vi "BLM_stepper motor V2.vi"() -> ()   [LabVIEW 2018]
doc: "To start rotations:\n\nSelect The Motor (BLM) address\nRun this VI\nClick Test connection button\nClick INITIALIZE button \n (It is assumed that a BLM controller should be initialized only once: immediately after it is turned on. \n E.g., usually there is no need to initialize if you rebooted computer, but kept the motor controller on,\n the motor was connected to the controller and you wish to continue using current position counting. \n Initialization occurs only if the current motor position is equal to zero.) \nClick READ BLM position button\nSelect desired MODE, SPEED, and Distance (or Final Position, depends on the MODE) value\nClick RUN BLM button\n\nSET POSITION button does not affect actual sample/motor position, but changes the position value\nin the controller memory. Thus, it allows to assign any value to the current motor position.\n\nSee also:\nhttps://opswiki.magnet.fsu.edu/wiki/pages/K7Q8u4C4s9/Rotating_probes_equipped_with_Brushless_Motors_BLMs.html\n\nNHMFL; A.Suslov; Feb 2012; updated Aug 2016"
uses:
  stepper motor action.ctl
  slider setter action.ctl
  stepper motor state.ctl
panel:
  in  "Tab Control":enum32{"main", "init&stuff", "ignore"}(tab)
  in  "stepper state":T1=enum."stopped"
  in  "set angle":dbl(slide)=-18.244680851063833 scale=-95.0..95.0 scale format="%^#6_6g"
  in  "XY Graph":cluster{dbl[], dbl[]}[](graph)=[{[-0.2849184585575504, -0.22366098996767705, -0.16240352137780373, -0.10114605278793037, -0.03988858419805705, 0.02136888439181628, 0.08262635298168963, 0.14388382157156293, 0.20514129016143628, 0.2663987587513096, 0.32765622734118294, 0.3889136959310563, 0.45017116452092965, 0.511428633110803, 0.5726861017006762, 0.6339435702905496, 0.695201038880423, 0.7564585074702963, 0.8177159760601695, 0.878973444650043], [0.09392269147117449, 0.07372931280487197, 0.053535934138569455, 0.03334255547226694, 0.013149176805964419, -0.007044201860338106, -0.027237580526640617, -0.04743095919294313, -0.06762433785924565, -0.08781771652554818, -0.1080110951918507, -0.1282044738581532, -0.14839785252445573, -0.16859123119075825, -0.18878460985706075, -0.2089779885233633, -0.2291713671896658, -0.2493647458559683, -0.26955812452227085, -0.28975150318857334]}, {[0.02614672282429747, 0.020525177417073513, 0.014903632009849559, 0.0092820866026256, 0.003660541195401646, -0.0019610042118223085, -0.00758254961904627, -0.013204095026270225, -0.01882564043349418, -0.024447185840718134, -0.03006873124794209, -0.03569027665516605, -0.04131182206239001, -0.04693336746961396, -0.05255491287683792, -0.05817645828406187, -0.06379800369128583, -0.06941954909850978, -0.07504109450573374, -0.08066263991295769], [0.2988584094275236, 0.23460385140060602, 0.17034929337368845, 0.10609473534677089, 0.04184017731985329, -0.022414380707064308, -0.08666893873398185, -0.15092349676089944, -0.21517805478781704, -0.27943261281473464, -0.34368717084165223, -0.40794172886856983, -0.4721962868954873, -0.5364508449224049, -0.6007054029493225, -0.6649599609762401, -0.7292145190031577, -0.7934690770300753, -0.8577236350569929, -0.9219781930839105]}, {[1.0, 0.9980267284282716, 0.9921147013144779, 0.9822872507286887, 0.9685831611286311, 0.9510565162951535, 0.9297764858882513, 0.9048270524660195, 0.8763066800438636, 0.8443279255020151, 0.8090169943749475, 0.7705132427757891, 0.7289686274214116, 0.6845471059286886, 0.6374239897486896, 0.587785252292473, 0.5358267949789965, 0.48175367410171516, 0.42577929156507266, 0.36812455268467786, 0.30901699437494745, 0.24868988716485474, 0.18738131458572452, 0.12533323356430426, 0.0627905195293133, -1.6081428723391245e-16, -0.0627905195293134, -0.12533323356430437, -0.18738131458572482, -0.24868988716485485, -0.30901699437494756, -0.368124552684678, -0.4257792915650727, -0.48175367410171543, -0.5358267949789969, -0.587785252292473, -0.6374239897486897, -0.6845471059286887, -0.7289686274214117, -0.7705132427757894, -0.8090169943749473, -0.8443279255020151, -0.8763066800438636, -0.9048270524660196, -0.9297764858882515, -0.9510565162951536, -0.9685831611286311, -0.9822872507286887, -0.9921147013144779, -0.9980267284282716, -1.0, -0.9980267284282716, -0.9921147013144779, -0.9822872507286886, -0.9685831611286311, -0.9510565162951535, -0.9297764858882512, -0.9048270524660195, -0.8763066800438635, -0.844327925502015, -0.8090169943749472, -0.770513242775789, -0.7289686274214116, -0.6845471059286886, -0.6374239897486895, -0.5877852522924732, -0.5358267949789963, -0.48175367410171527, -0.42577929156507216, -0.3681245526846778, -0.30901699437494756, -0.24868988716485443, -0.18738131458572463, -0.12533323356430373, -0.06279051952931321, -1.836909530733566e-16, 0.06279051952931372, 0.12533323356430423, 0.18738131458572513, 0.24868988716485493, 0.30901699437494723, 0.36812455268467825, 0.4257792915650726, 0.4817536741017157, 0.5358267949789968, 0.5877852522924737, 0.63742398974869, 0.6845471059286886, 0.7289686274214119, 0.7705132427757894, 0.8090169943749478, 0.8443279255020153, 0.8763066800438636, 0.9048270524660197, 0.9297764858882515, 0.9510565162951538, 0.9685831611286312, 0.9822872507286887, 0.9921147013144779, 0.9980267284282716], [0.0, 0.06279051952931337, 0.12533323356430426, 0.18738131458572463, 0.2486898871648548, 0.3090169943749474, 0.368124552684678, 0.4257792915650727, 0.4817536741017153, 0.5358267949789967, 0.5877852522924731, 0.6374239897486897, 0.6845471059286887, 0.7289686274214116, 0.7705132427757893, 0.8090169943749475, 0.8443279255020151, 0.8763066800438637, 0.9048270524660196, 0.9297764858882515, 0.9510565162951535, 0.9685831611286311, 0.9822872507286887, 0.9921147013144779, 0.9980267284282716, 1.0, 0.9980267284282716, 0.9921147013144778, 0.9822872507286886, 0.9685831611286311, 0.9510565162951535, 0.9297764858882513, 0.9048270524660195, 0.8763066800438635, 0.844327925502015, 0.8090169943749475, 0.7705132427757893, 0.7289686274214114, 0.6845471059286885, 0.6374239897486895, 0.5877852522924732, 0.5358267949789967, 0.4817536741017152, 0.4257792915650725, 0.36812455268467775, 0.3090169943749471, 0.24868988716485482, 0.18738131458572457, 0.1253332335643041, 0.06279051952931314, -3.216285744678249e-16, -0.06279051952931335, -0.12533323356430429, -0.18738131458572477, -0.24868988716485502, -0.30901699437494773, -0.3681245526846783, -0.42577929156507266, -0.4817536741017154, -0.5358267949789968, -0.5877852522924734, -0.63742398974869, -0.6845471059286887, -0.7289686274214116, -0.7705132427757894, -0.8090169943749473, -0.8443279255020153, -0.8763066800438636, -0.9048270524660198, -0.9297764858882515, -0.9510565162951535, -0.9685831611286312, -0.9822872507286887, -0.9921147013144779, -0.9980267284282716, -1.0, -0.9980267284282716, -0.9921147013144779, -0.9822872507286886, -0.9685831611286311, -0.9510565162951536, -0.9297764858882512, -0.9048270524660196, -0.8763066800438634, -0.844327925502015, -0.809016994374947, -0.770513242775789, -0.7289686274214116, -0.6845471059286883, -0.6374239897486896, -0.5877852522924726, -0.5358267949789963, -0.4817536741017153, -0.4257792915650722, -0.36812455268467786, -0.3090169943749468, -0.2486898871648545, -0.18738131458572468, -0.1253332335643038, -0.06279051952931326]}, {[0.1, 0.09980267284282716, 0.0992114701314478, 0.09822872507286888, 0.09685831611286311, 0.09510565162951536, 0.09297764858882514, 0.09048270524660196, 0.08763066800438636, 0.08443279255020152, 0.08090169943749476, 0.07705132427757892, 0.07289686274214116, 0.06845471059286887, 0.06374239897486897, 0.05877852522924731, 0.05358267949789966, 0.04817536741017152, 0.042577929156507266, 0.03681245526846779, 0.030901699437494747, 0.024868988716485477, 0.018738131458572452, 0.012533323356430426, 0.006279051952931331, -1.6081428723391246e-17, -0.0062790519529313405, -0.012533323356430438, -0.018738131458572484, -0.024868988716485487, -0.030901699437494757, -0.0368124552684678, -0.04257792915650727, -0.048175367410171546, -0.05358267949789969, -0.05877852522924731, -0.06374239897486898, -0.06845471059286888, -0.07289686274214117, -0.07705132427757894, -0.08090169943749474, -0.08443279255020152, -0.08763066800438636, -0.09048270524660196, -0.09297764858882515, -0.09510565162951537, -0.09685831611286311, -0.09822872507286888, -0.0992114701314478, -0.09980267284282716, -0.1, -0.09980267284282716, -0.0992114701314478, -0.09822872507286887, -0.09685831611286311, -0.09510565162951536, -0.09297764858882512, -0.09048270524660196, -0.08763066800438635, -0.0844327925502015, -0.08090169943749473, -0.07705132427757891, -0.07289686274214116, -0.06845471059286887, -0.06374239897486896, -0.05877852522924733, -0.05358267949789963, -0.04817536741017153, -0.04257792915650722, -0.036812455268467784, -0.030901699437494757, -0.024868988716485445, -0.018738131458572463, -0.012533323356430374, -0.006279051952931321, -1.836909530733566e-17, 0.006279051952931373, 0.012533323356430424, 0.018738131458572515, 0.024868988716485494, 0.030901699437494726, 0.036812455268467825, 0.042577929156507266, 0.048175367410171574, 0.05358267949789968, 0.05877852522924737, 0.063742398974869, 0.06845471059286887, 0.07289686274214119, 0.07705132427757894, 0.08090169943749478, 0.08443279255020153, 0.08763066800438636, 0.09048270524660197, 0.09297764858882515, 0.09510565162951538, 0.09685831611286312, 0.09822872507286888, 0.0992114701314478, 0.09980267284282716], [0.0, 0.006279051952931338, 0.012533323356430426, 0.018738131458572463, 0.02486898871648548, 0.03090169943749474, 0.0368124552684678, 0.04257792915650727, 0.04817536741017153, 0.05358267949789967, 0.058778525229247314, 0.06374239897486898, 0.06845471059286888, 0.07289686274214116, 0.07705132427757894, 0.08090169943749476, 0.08443279255020152, 0.08763066800438638, 0.09048270524660196, 0.09297764858882515, 0.09510565162951536, 0.09685831611286311, 0.09822872507286888, 0.0992114701314478, 0.09980267284282716, 0.1, 0.09980267284282716, 0.09921147013144778, 0.09822872507286887, 0.09685831611286311, 0.09510565162951536, 0.09297764858882514, 0.09048270524660196, 0.08763066800438635, 0.0844327925502015, 0.08090169943749476, 0.07705132427757894, 0.07289686274214115, 0.06845471059286885, 0.06374239897486896, 0.05877852522924733, 0.05358267949789967, 0.048175367410171525, 0.04257792915650725, 0.03681245526846778, 0.030901699437494712, 0.024868988716485484, 0.01873813145857246, 0.01253332335643041, 0.0062790519529313145, -3.216285744678249e-17, -0.006279051952931335, -0.01253332335643043, -0.018738131458572477, -0.024868988716485504, -0.030901699437494774, -0.03681245526846783, -0.042577929156507266, -0.04817536741017154, -0.05358267949789968, -0.05877852522924734, -0.063742398974869, -0.06845471059286888, -0.07289686274214116, -0.07705132427757894, -0.08090169943749474, -0.08443279255020153, -0.08763066800438636, -0.09048270524660199, -0.09297764858882515, -0.09510565162951536, -0.09685831611286312, -0.09822872507286888, -0.0992114701314478, -0.09980267284282716, -0.1, -0.09980267284282716, -0.0992114701314478, -0.09822872507286887, -0.09685831611286311, -0.09510565162951537, -0.09297764858882512, -0.09048270524660196, -0.08763066800438635, -0.0844327925502015, -0.0809016994374947, -0.07705132427757891, -0.07289686274214116, -0.06845471059286883, -0.06374239897486897, -0.05877852522924726, -0.05358267949789963, -0.04817536741017153, -0.042577929156507224, -0.03681245526846779, -0.03090169943749468, -0.02486898871648545, -0.01873813145857247, -0.012533323356430379, -0.006279051952931327]}, {[0.0, 0.0, 0.0, 0.0, 0.0, 0.0, 0.0, 0.0, 0.0, 0.0, 0.0, 0.0, 0.0, 0.0, 0.0, 0.0, 0.0, 0.0, 0.0, 0.0], [1.1, 1.135, 1.1700000000000002, 1.205, 1.24, 1.2750000000000001, 1.31, 1.345, 1.3800000000000001, 1.415, 1.4500000000000002, 1.485, 1.52, 1.5550000000000002, 1.59, 1.625, 1.6600000000000001, 1.695, 1.73, 1.7650000000000001]}, {[6.735334946023075e-17, 6.796565263714194e-17, 6.857795581405312e-17, 6.919025899096432e-17, 6.980256216787551e-17, 7.04148653447867e-17, 7.102716852169788e-17, 7.163947169860908e-17, 7.225177487552027e-17, 7.286407805243145e-17, 7.347638122934264e-17, 7.408868440625383e-17, 7.470098758316503e-17, 7.53132907600762e-17, 7.59255939369874e-17, 7.653789711389858e-17, 7.715020029080977e-17, 7.776250346772096e-17, 7.837480664463216e-17, 7.898710982154334e-17], [1.1, 1.11, 1.12, 1.1300000000000001, 1.1400000000000001, 1.1500000000000001, 1.1600000000000001, 1.1700000000000002, 1.1800000000000002, 1.1900000000000002, 1.2000000000000002, 1.21, 1.22, 1.23, 1.24, 1.25, 1.26, 1.27, 1.28, 1.29]}, {[-0.09587131702242406, -0.09674287444990064, -0.09761443187737723, -0.0984859893048538, -0.0993575467323304, -0.10022910415980697, -0.10110066158728355, -0.10197221901476014, -0.10284377644223672, -0.10371533386971331, -0.10458689129718989, -0.10545844872466646, -0.10633000615214305, -0.10720156357961963, -0.10807312100709622, -0.1089446784345728, -0.10981623586204937, -0.11068779328952597, -0.11155935071700254, -0.11243090814447912], [-1.0958141679009201, -1.1057761148818375, -1.115738061862755, -1.1257000088436726, -1.13566195582459, -1.1456239028055073, -1.1555858497864249, -1.1655477967673424, -1.1755097437482598, -1.1854716907291771, -1.1954336377100947, -1.2053955846910123, -1.2153575316719296, -1.225319478652847, -1.2352814256337645, -1.245243372614682, -1.2552053195955994, -1.2651672665765168, -1.2751292135574344, -1.285091160538352]}]
  out "cur angle":dbl(slide)=-95.0 scale=-95.0..95.0 scale format="%^#6_6g"
  in  "set step !":dbl(slide)=6845.744680851064 min=0.0 max=16000.0 scale=0.0..16500.0 scale format="%^#6_6g"
  out "cur step":dbl(slide) scale=0.0..16500.0
  in  "Go!":bool
  in  "Stop!":bool
  in  "set speed!":i32=2500
  out "Moving..":bool
  out "error out":errorcluster
  out "Current Bottom Position":dbl format="%.4f"
  in  "Move to Bottom Position (deg or in)":dbl=95.83933701824397 format="%.4f"
  in  "Rotator":T2(ring)=enum."System B 50 mm Magnet"
  out "Timeout error":bool
  in  "Motor Address":string="0"
  out "Error Out":errorcluster {"code" format="%.0x"}
  in  "MODE:":enum32{"ABSOLUTE", "INCREMENTAL"}(radio)=enum."INCREMENTAL"
  in  "Read Position":bool
  out "Test Results":string
  in  "Test Connection":bool
  out "BLM Position":dbl caption="BLM position\nincrement 0.045 \n (deg of BLM)" format="%.3f"
  in  "Parameter changed":bool
  in  "stop":bool
  in  "Set Position":bool
  in  "INITIALIZE":bool
  in  "Run":bool
  in  "New position":dbl caption="Final position:\nincrement 0.045 \n (deg of BLM)" step=0.045 format="%#.3g"
  in  "SPEED (rot/sec)\nincrement .0042":dbl=0.0294 min=0.0042 max=0.42 step=0.0042
  in  "MOTOR (BLM) Address":refnum<visa-resource-name>
  # "Select The Motor (BLM) address\nRun this VI\nClick Test connection button\nClick  INITIALIZE button \nClick  READ BLM position button\nSelect desired MODE, SPEED, and\n         Distance (or Final Position)\nClick RUN BLM button\n\nMore Help at File-> VI Propeties->\nDocumentation\nand Operations Wiki"
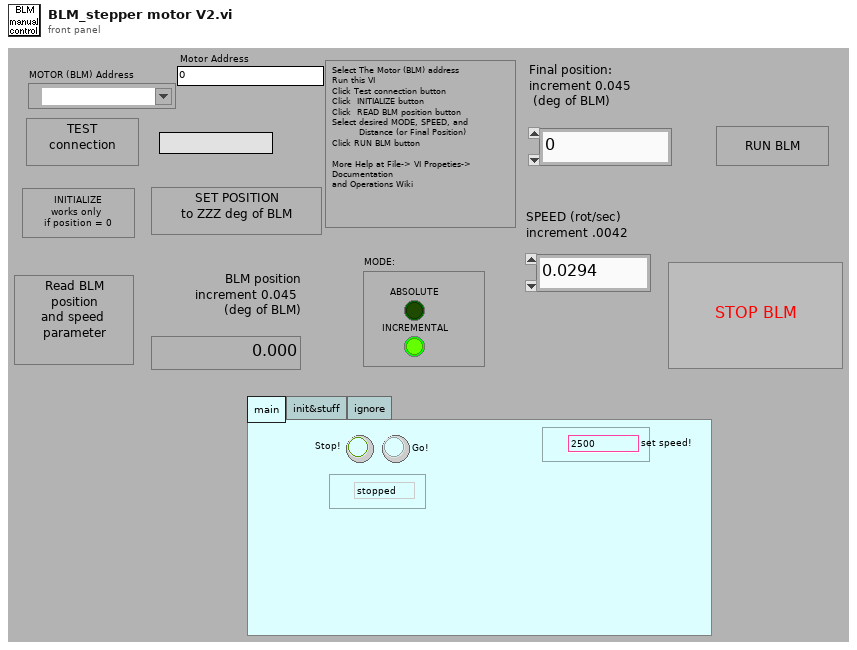
[diagram p1: front panel]
types:
  T1 = typedef "stepper motor state.ctl" = enum16{"moving", "stopped"}
  T2 = enum16{"Dilution Fridge SCM 1", "System A SCM 2", "System B 50 mm Magnet", "He-3 32 mm Magnet", "Portable Dil Fridge Rotator", "Linear Position", "System E Probe 1"}
  T3 = typedef "stepper motor action.ctl" = enum16{"go", "void", "stop", "check", "init", "sync", "set", "set speed"}
  T4 = enum8{"Enabled", "Disabled", "Disabled and Grayed Out"}
  T5 = typedef "slider setter action.ctl" = enum16{"--update circle", "set step slider moves", "cursor moves", "current pos changed", "init", "void", "--draw current lie", "--draw set line", "--move current step slider", "--move set step slider", "--draw limit lines", "check", "--move set angle slider", "--move current angle slider", "set angle slider moves", "--move cursor", "set set step", "set current step"}
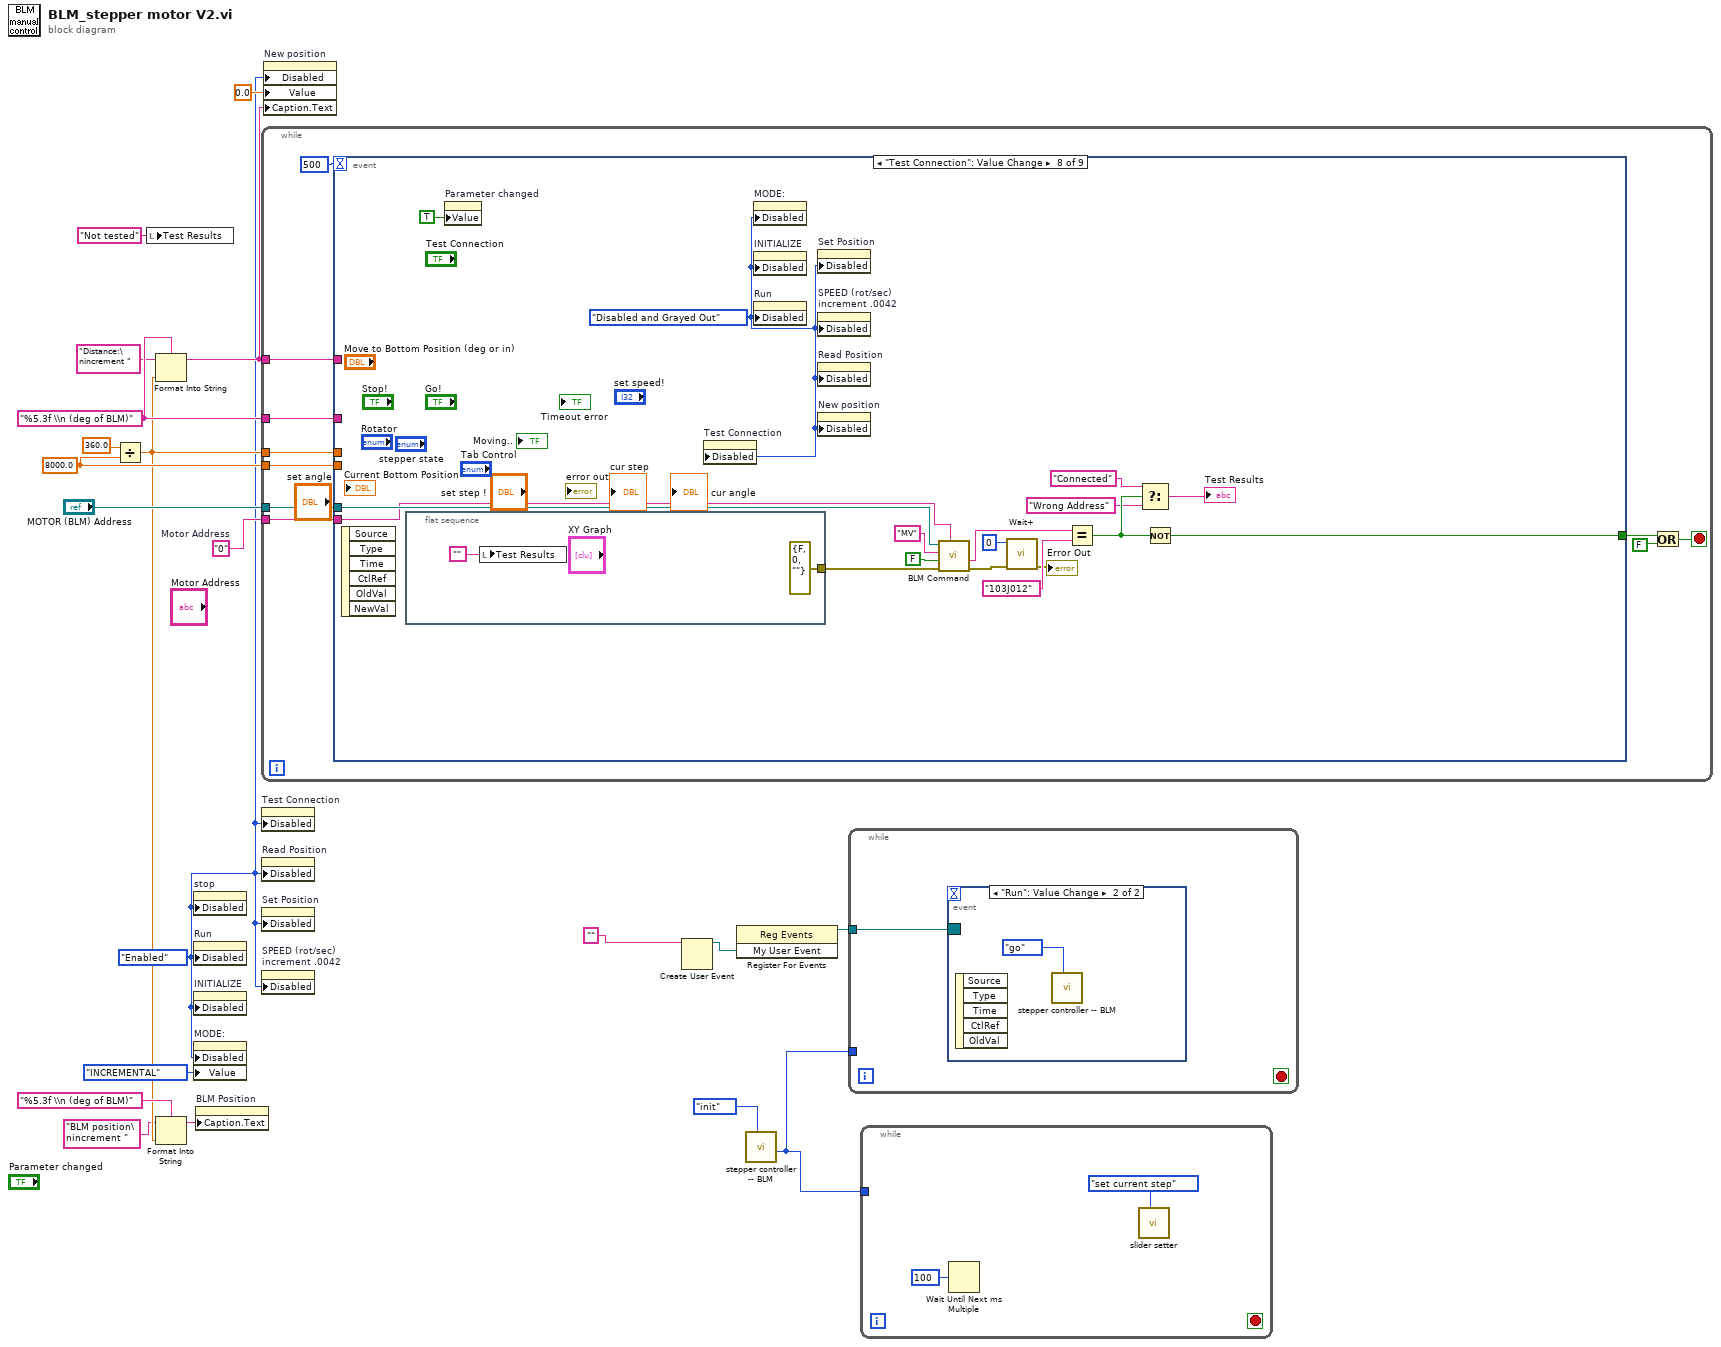
[diagram p0: block diagram]
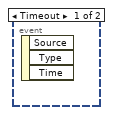
[diagram p2: hidden frame]
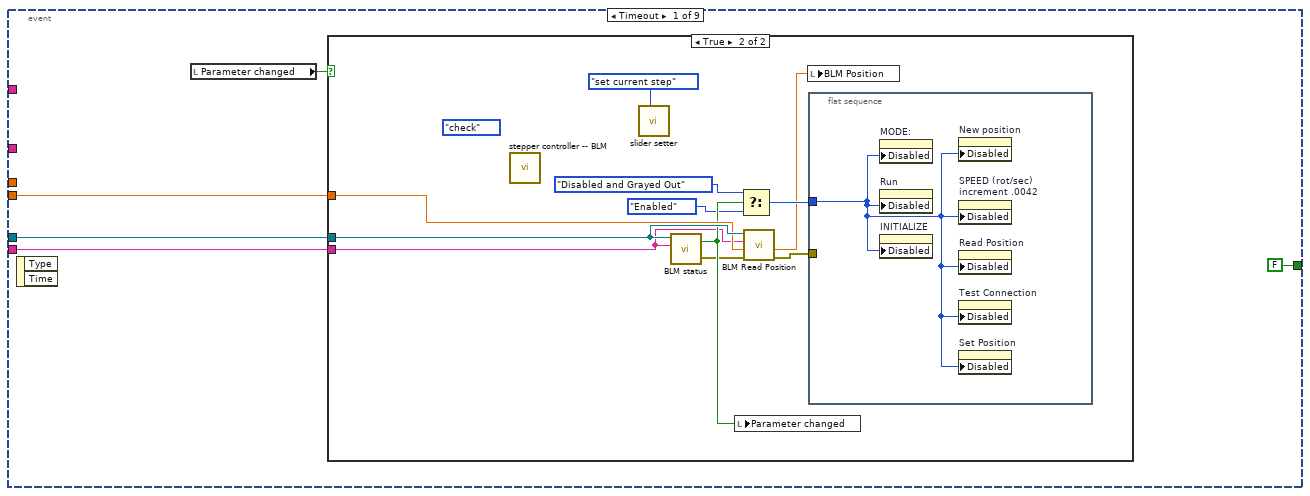
[diagram p3: hidden frame]
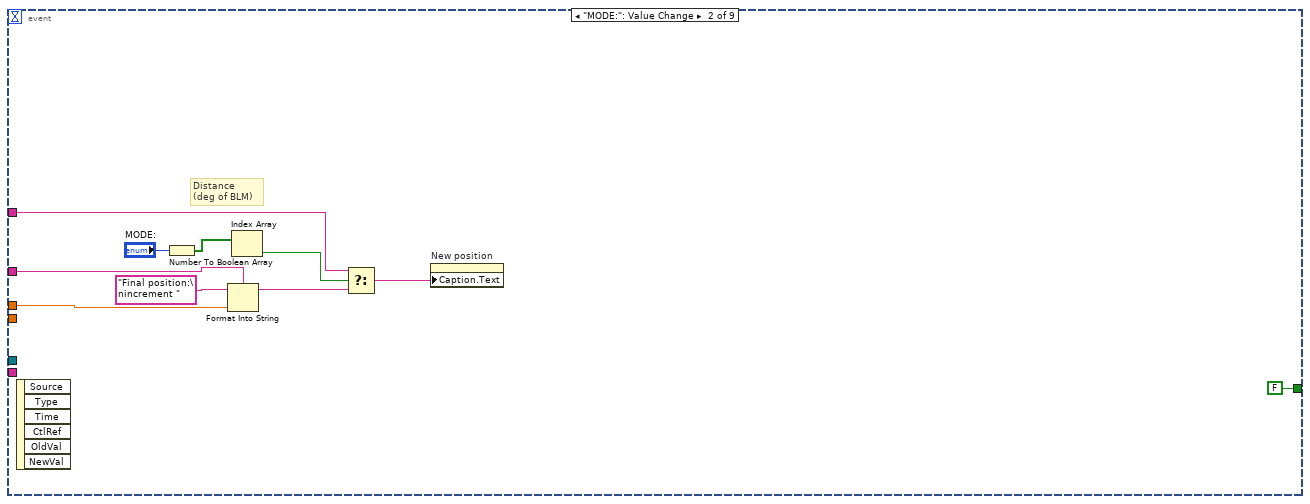
[diagram p5: hidden frame]
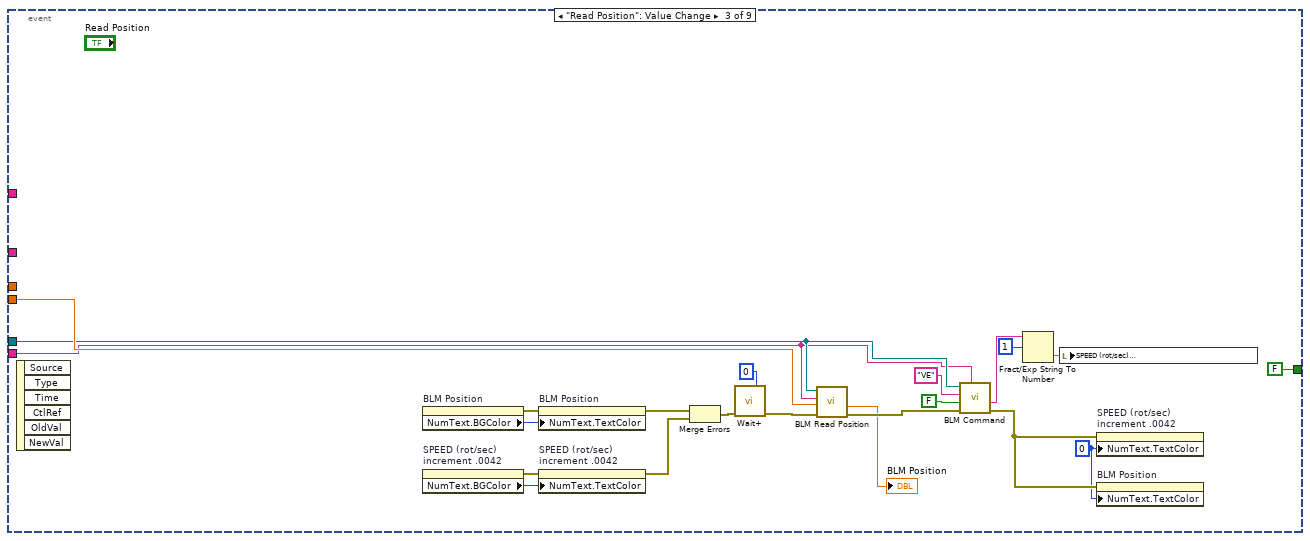
[diagram p6: hidden frame]
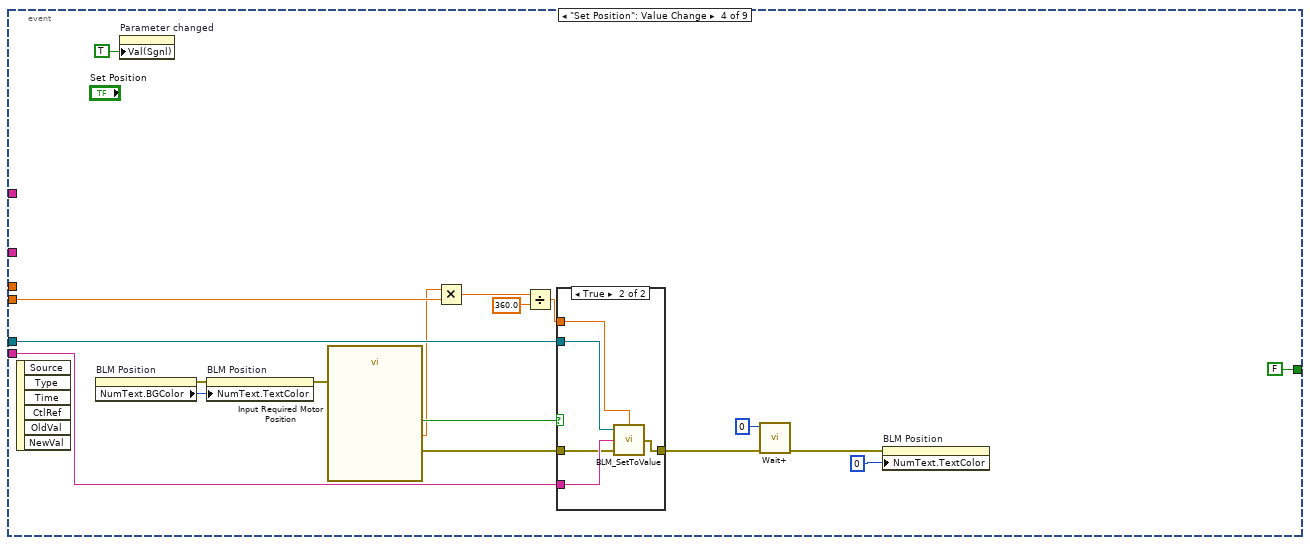
[diagram p7: hidden frame]
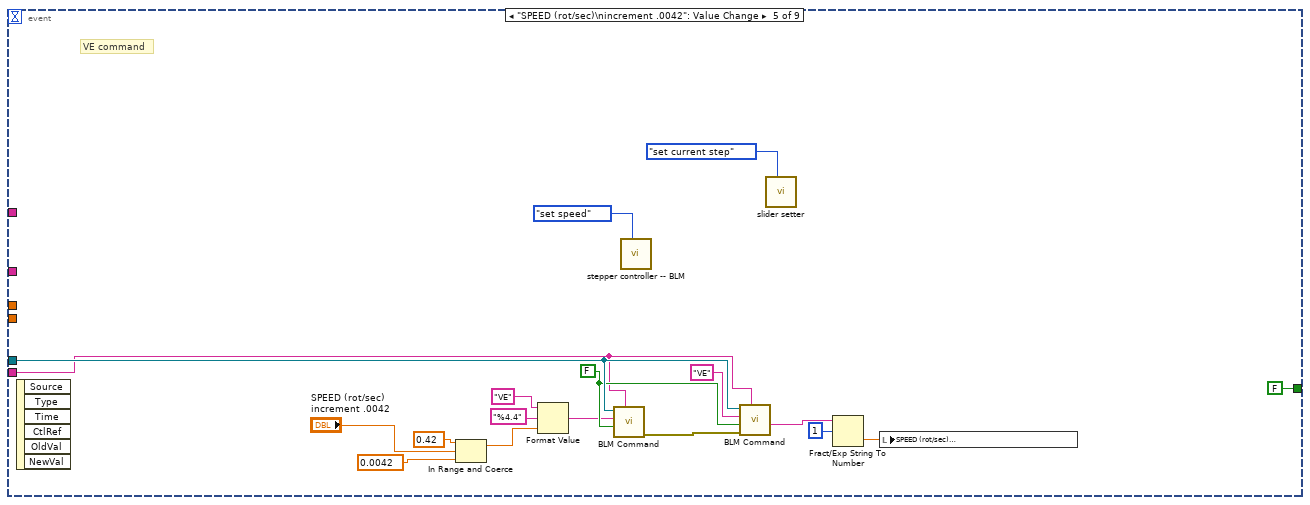
[diagram p9: hidden frame]
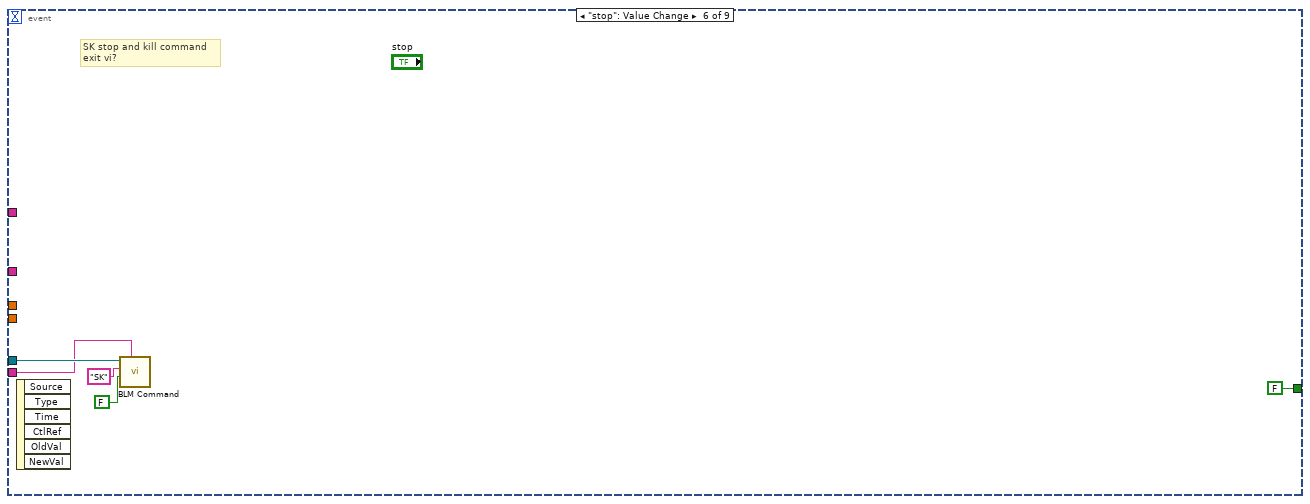
[diagram p10: hidden frame]
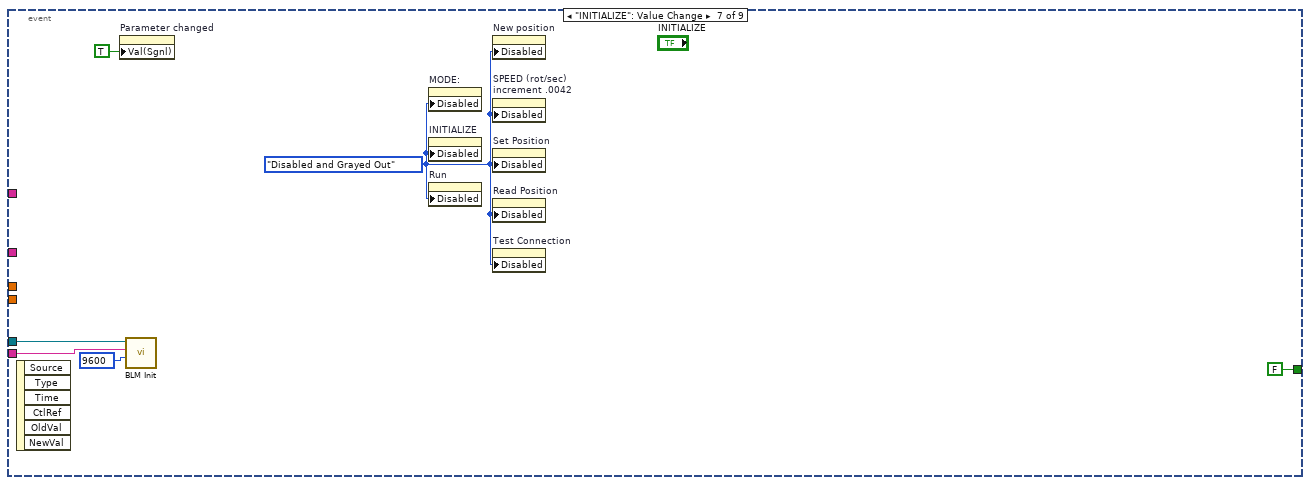
[diagram p11: hidden frame]
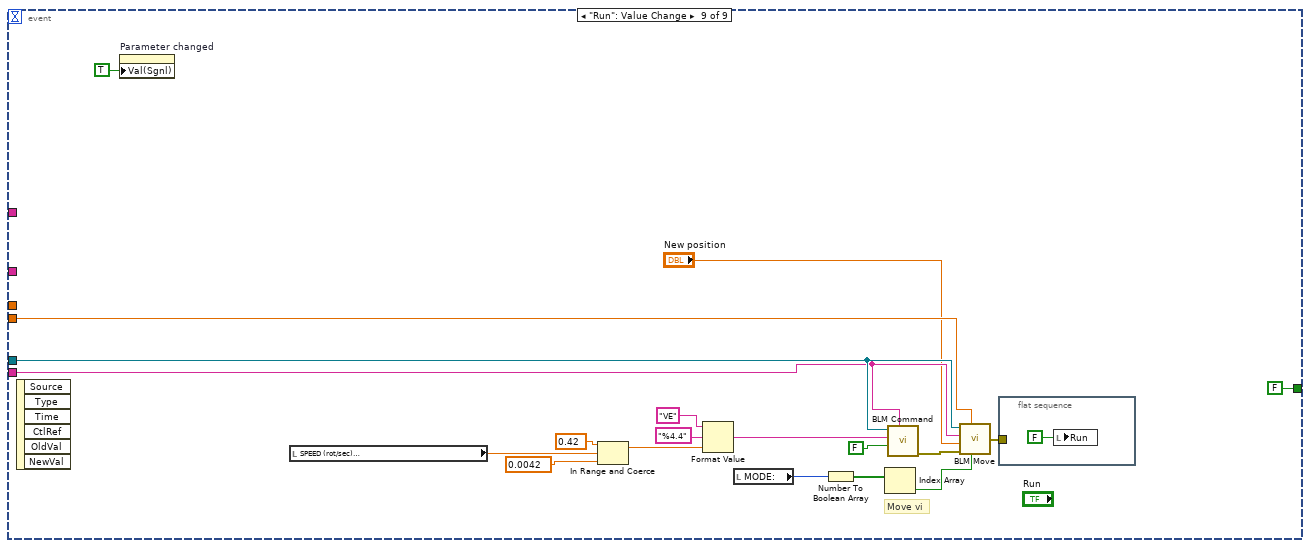
[diagram p12: hidden frame]
diagram:
  w7 = T4."Enabled" ("Disabled")
  w13 = "%5.3f \\n (deg of BLM)" ("format string")
  w17 = "0"  # Motor Address
  w15 = 8000.0 ("Steps/rot")
  n1 = Divide(x=360.0, y=w15) -> (x/y=w10:dbl)
  n2 = local write "Test Results"("Not tested" ("s? t:f")) -> ()
  n3 = Format Into String(format string=w13, initial string="Distance:\nincrement " ("Label.Text"), w10) -> (resulting string=w14:string)  [unwired: 1 in, 1 out]
  n4 = Format Into String(format string="%5.3f \\n (deg of BLM)", initial string="BLM position\nincrement ", w10) -> (resulting string=w11:string)  [unwired: 1 in, 1 out]
  n5 = property on="stop" class="Bool"("Disabled"=w7) -> ()  [unwired: 2 in, 2 out]
  n6 = property on="Run" class="Bool (strict)"("Disabled"=w7) -> ()  [unwired: 2 in, 2 out]
  n7 = property on="INITIALIZE" class="Bool"("Disabled"=w7) -> ()  [unwired: 2 in, 2 out]
  n8 = property on="MODE:" class="RadioBtnsControl (strict)"("Disabled"=w7, "Value"=enum32{"ABSOLUTE", "INCREMENTAL"}."INCREMENTAL" ("MODE:")) -> ()  [unwired: 2 in, 2 out]
  n9 = property on="BLM Position" class="DigNum (strict)"("Caption.Text"=w11) -> ()  [unwired: 2 in, 2 out]
  n10 = while {
    tunnel: w15 -> [w30]
    tunnel: "MOTOR (BLM) Address" -> [w29]
    tunnel: w14 -> [w24]
    tunnel: w17 -> [w23]
    tunnel: w10 -> [w22]
    tunnel: w13 -> [w21]
    stop <- w26 stop-if-true
    n11 = event shown="[7] \"Test Connection\": Value Change" {
      selector: _ -> [_ _ _ _ _ _ _ _ _]
      dyn-events: _ -> [_ _ _ _ _ _ _ _ _]
      timeout: 500 -> [_ _ _ _ _ _ _ _ _]
      tunnel: w30 -> [w34 _ w79 w94 _ _ _ _ w170]
      tunnel: w29 -> [w35 _ w78 w97 w121 w126 w131 w149 w169]
      tunnel: [FALSE FALSE FALSE FALSE FALSE FALSE FALSE w147 FALSE] -> w25
      tunnel: w24 -> [_ w56 _ _ _ _ _ _ _]
      tunnel: w23 -> [w32 _ w77 w95 w117 w123 w129 w145 w167]
      tunnel: w22 -> [_ w50 _ _ _ _ _ _ _]
      tunnel: w21 -> [_ w49 _ _ _ _ _ _ _]
      event Timeout {
        n12 = event-data() -> ()  [unwired: 1 in, 2 out]
        n13 = local read "Parameter changed"() -> (w33:bool)
        n14 = case shown="True" w33 {
          tunnel: w35 -> [_ w46]
          tunnel: w34 -> [_ w45]
          tunnel: w32 -> [_ w41]
          frame False {
          }
          frame True {
            (unwired) stepper_motor_action."check" ("stepper motor action")
            n15 = call "stepper controller -- BLM.vi"() -> ()  [unwired: 9 in, 3 out]
            n16 = call "slider setter.vi"("slider setter action"=slider_setter_action."set current step") -> ()  [unwired: 10 in, 1 out]
            n17 = call "BLM status.vi"("Motor Address"=w41, "Porty Address"=w46) -> ("error out"=w40:errorcluster, "Motor is moving"=w44:bool)  [unwired: 2 in]
            n18 = local write "Parameter changed"(w44) -> ()
            n19 = Select(t=T4."Disabled and Grayed Out" ("Disabled"), s=w44, f=T4."Enabled" ("Disabled")) -> (s? t:f=w43:T4)
            n20 = call "BLM Read Position.vi"("error in (no error)"=w40, "Steps/rot"=w45, "Motor Address"=w41, "Port Address"=w46) -> ("error out"=w39:errorcluster, "Response"=w42:dbl)  [unwired: 2 out]
            n21 = local write "BLM Position"(w42) -> ()
            n22 = flat-sequence {
              tunnel: w43 -> [w47]
              tunnel: w39 -> [_]
              frame #0 {
                n23 = property on="MODE:" class="RadioBtnsControl (strict)"("Disabled"=w47) -> ()  [unwired: 2 in, 2 out]
                n24 = property on="Run" class="Bool (strict)"("Disabled"=w47) -> ()  [unwired: 2 in, 2 out]
                n25 = property on="INITIALIZE" class="Bool"("Disabled"=w47) -> ()  [unwired: 2 in, 2 out]
                n26 = property on="New position" class="DigNum (strict)"("Disabled"=w47) -> ()  [unwired: 2 in, 2 out]
                n27 = property on="SPEED (rot/sec)\nincrement .0042" class="DigNum (strict)"("Disabled"=w47) -> ()  [unwired: 2 in, 2 out]
                n28 = property on="Read Position" class="Bool"("Disabled"=w47) -> ()  [unwired: 2 in, 2 out]
                n29 = property on="Test Connection" class="Bool"("Disabled"=w47) -> ()  [unwired: 2 in, 2 out]
                n30 = property on="Set Position" class="Bool"("Disabled"=w47) -> ()  [unwired: 2 in, 2 out]
              }
            }
          }
        }
      }
      event "MODE:": Value Change {
        # "Distance  \n(deg of BLM)"
        n31 = event-data() -> ()  [unwired: 1 in, 6 out]
        n32 = Number To Boolean Array(number="MODE:") -> (Boolean array=w54:bool[])
        n33 = Format Into String(format string=w49, initial string="Final position:\nincrement " ("f"), w50) -> (resulting string=w52:string)  [unwired: 1 in, 1 out]
        n34 = Index Array(array=w54) -> (element=w53:bool)  [unwired: 1 in]
        n35 = Select(t=w56, s=w53, f=w52) -> (s? t:f=w57:string)
        n36 = property on="New position" class="DigNum (strict)"("Caption.Text"=w57) -> ()  [unwired: 2 in, 2 out]
      }
      event "Read Position": Value Change {
        w64 = u32 0 ("Numeric Text.Text Colors:Text Color")
        n37 = event-data() -> ()  [unwired: 1 in, 6 out]
        n38 = property on="BLM Position" class="DigNum (strict)"() -> (error out=w58:errorcluster, "NumText.BGColor"=w63:u32)  [unwired: 2 in, 1 out]
        n39 = property on="SPEED (rot/sec)\nincrement .0042" class="DigNum (strict)"() -> (error out=w59:errorcluster, "NumText.BGColor"=w62:u32)  [unwired: 2 in, 1 out]
        n40 = property on="BLM Position" class="DigNum (strict)"(error in=w58, "NumText.TextColor"=w63) -> (error out=w61:errorcluster)  [unwired: 1 in, 1 out]
        n41 = property on="SPEED (rot/sec)\nincrement .0042" class="DigNum (strict)"(error in=w59, "NumText.TextColor"=w62) -> (error out=w60:errorcluster)  [unwired: 1 in, 1 out]
        n42 = Merge Errors(w61, w60) -> (w65:errorcluster)
        n43 = call "Wait+.vi"("Error In"=w65, "milliseconds to wait"=u32 0 ("millisecond timer value")) -> ("Error Out"=w67:errorcluster)  [unwired: 4 in, 1 out]
        n44 = call "BLM Read Position.vi"("error in (no error)"=w67, "Steps/rot"=w79, "Motor Address"=w77, "Port Address"=w78) -> ("error out"=w69:errorcluster, "Response"=→"BLM Position":dbl)  [unwired: 2 out]
        n45 = call "BLM Command.vi"("Motor Address"=w77, "error in (no error)"=w69, "Read Echo?"=FALSE, "Command"="VE", "Port Address"=w78) -> ("error out"=w75:errorcluster, "Response"=w72:string)  [unwired: 1 in, 3 out]
        n46 = Fract/Exp String To Number(string=w72, offset=1) -> (number=w70:dbl)  [unwired: 2 in, 1 out]
        n47 = local write "SPEED (rot/sec)\nincrement .0042"(w70) -> ()
        n48 = property on="SPEED (rot/sec)\nincrement .0042" class="DigNum (strict)"(error in=w75, "NumText.TextColor"=w64) -> ()  [unwired: 1 in, 2 out]
        n49 = property on="BLM Position" class="DigNum (strict)"(error in=w75, "NumText.TextColor"=w64) -> ()  [unwired: 1 in, 2 out]
      }
      event "Set Position": Value Change {
        n50 = event-data() -> ()  [unwired: 1 in, 6 out]
        n51 = property on="BLM Position" class="DigNum (strict)"() -> (error out=w80:errorcluster, "NumText.BGColor"=w89:u32)  [unwired: 2 in, 1 out]
        n52 = property on="Parameter changed" class="Bool (strict)"("Val(Sgnl)"=TRUE ("Value (Signaling)")) -> ()  [unwired: 2 in, 2 out]
        n53 = property on="BLM Position" class="DigNum (strict)"(error in=w80, "NumText.TextColor"=w89) -> (error out=w90:errorcluster)  [unwired: 1 in, 1 out]
        n54 = call "Input Required Motor Position"("error in (no error)"=w90) -> ("Position:"=w87:dbl, "OK"=w88:bool, "error out"=w83:errorcluster)  [unwired: 16 in]
        n55 = Multiply(x=w87, y=w94) -> (x*y=w85:dbl)
        n56 = Divide(x=w85, y=360.0) -> (x/y=w86:dbl)
        n57 = case shown="True" w88 {
          tunnel: w97 -> [_ w103]
          tunnel: w95 -> [_ w102]
          tunnel: w86 -> [_ w101]
          tunnel: [w98 w100] -> w92
          tunnel: w83 -> [w98 w99]
          frame False {
          }
          frame True {
            n58 = call "BLM_SetToValue.vi"("Position"=w101, "error in (no error)"=w99, "Motor Address"=w102, "Port Address"=w103) -> ("error out"=w100:errorcluster)
          }
        }
        n59 = call "Wait+.vi"("Error In"=w92, "milliseconds to wait"=u32 0) -> ("Error Out"=w91:errorcluster)  [unwired: 4 in, 1 out]
        n60 = property on="BLM Position" class="DigNum (strict)"(error in=w91, "NumText.TextColor"=u32 0 ("Numeric Text.Text Colors:Text Color")) -> ()  [unwired: 1 in, 2 out]
      }
      event "SPEED (rot/sec)\nincrement .0042": Value Change {
        w120 = FALSE
        # "VE command"
        n61 = event-data() -> ()  [unwired: 1 in, 6 out]
        n62 = In Range and Coerce(upper limit=0.42 ("x"), x="SPEED (rot/sec)\nincrement .0042", lower limit=0.0042) -> (coerced(x)=w113:dbl)  [unwired: 1 out]
        n63 = Format Value(string ("")="VE", format string="%4.4", value (0)=w113) -> (output string=w110:string)
        n64 = call "BLM Command.vi"("Motor Address"=w117, "Read Echo?"=w120, "Command"=w110, "Port Address"=w121) -> ("error out"=w118:errorcluster)  [unwired: 2 in, 4 out]
        n65 = call "stepper controller -- BLM.vi"("stepper driver action"=stepper_motor_action."set speed" ("stepper motor action")) -> ()  [unwired: 8 in, 3 out]
        n66 = call "BLM Command.vi"("Motor Address"=w117, "error in (no error)"=w118, "Read Echo?"=w120, "Command"="VE", "Port Address"=w121) -> ("Response"=w107:string)  [unwired: 1 in, 4 out]
        n67 = call "slider setter.vi"("slider setter action"=slider_setter_action."set current step") -> ()  [unwired: 10 in, 1 out]
        n68 = Fract/Exp String To Number(string=w107, offset=1) -> (number=w119:dbl)  [unwired: 2 in, 1 out]
        n69 = local write "SPEED (rot/sec)\nincrement .0042"(w119) -> ()
      }
      event "stop": Value Change {
        # "SK stop and kill command\nexit vi?"
        n70 = event-data() -> ()  [unwired: 1 in, 6 out]
        n71 = call "BLM Command.vi"("Motor Address"=w123, "Read Echo?"=FALSE, "Command"="SK", "Port Address"=w126) -> ()  [unwired: 2 in, 5 out]
      }
      event "INITIALIZE": Value Change {
        w127 = T4."Disabled and Grayed Out" ("Disabled")
        n72 = event-data() -> ()  [unwired: 1 in, 6 out]
        n73 = property on="Parameter changed" class="Bool (strict)"("Val(Sgnl)"=TRUE ("Value (Signaling)")) -> ()  [unwired: 2 in, 2 out]
        n74 = call "BLM Init.vi"("Baud Rate"=u32 9600, "Motor Address"=w129, "Port Address"=w131) -> ()  [unwired: 1 in, 3 out]
        n75 = property on="MODE:" class="RadioBtnsControl (strict)"("Disabled"=w127) -> ()  [unwired: 2 in, 2 out]
        n76 = property on="INITIALIZE" class="Bool"("Disabled"=w127) -> ()  [unwired: 2 in, 2 out]
        n77 = property on="Run" class="Bool (strict)"("Disabled"=w127) -> ()  [unwired: 2 in, 2 out]
        n78 = property on="New position" class="DigNum (strict)"("Disabled"=w127) -> ()  [unwired: 2 in, 2 out]
        n79 = property on="SPEED (rot/sec)\nincrement .0042" class="DigNum (strict)"("Disabled"=w127) -> ()  [unwired: 2 in, 2 out]
        n80 = property on="Set Position" class="Bool"("Disabled"=w127) -> ()  [unwired: 2 in, 2 out]
        n81 = property on="Read Position" class="Bool"("Disabled"=w127) -> ()  [unwired: 2 in, 2 out]
        n82 = property on="Test Connection" class="Bool"("Disabled"=w127) -> ()  [unwired: 2 in, 2 out]
      }
      event "Test Connection": Value Change {
        w144 = T4."Disabled and Grayed Out" ("Disabled")
        n83 = event-data() -> ()  [unwired: 1 in, 6 out]
        n84 = flat-sequence {
          tunnel: [errorcluster {"status"=FALSE, "code"=0, "source"=""} ("error in (no error)")] -> w134
          frame #0 {
            n85 = local write "Test Results"("" ("Response")) -> ()
          }
        }
        n86 = property on="Parameter changed" class="Bool (strict)"("Value"=TRUE ("Parameter changed")) -> ()  [unwired: 2 in, 2 out]
        n87 = property on="Test Connection" class="Bool"("Disabled"=w144) -> ()  [unwired: 2 in, 2 out]
        n88 = property on="MODE:" class="RadioBtnsControl (strict)"("Disabled"=w144) -> ()  [unwired: 2 in, 2 out]
        n89 = property on="INITIALIZE" class="Bool"("Disabled"=w144) -> ()  [unwired: 2 in, 2 out]
        n90 = property on="Run" class="Bool (strict)"("Disabled"=w144) -> ()  [unwired: 2 in, 2 out]
        n91 = property on="Set Position" class="Bool"("Disabled"=w144) -> ()  [unwired: 2 in, 2 out]
        n92 = property on="SPEED (rot/sec)\nincrement .0042" class="DigNum (strict)"("Disabled"=w144) -> ()  [unwired: 2 in, 2 out]
        n93 = property on="Read Position" class="Bool"("Disabled"=w144) -> ()  [unwired: 2 in, 2 out]
        n94 = property on="New position" class="DigNum (strict)"("Disabled"=w144) -> ()  [unwired: 2 in, 2 out]
        n95 = call "BLM Command.vi"("Motor Address"=w145, "error in (no error)"=w134, "Read Echo?"=FALSE, "Command"="MV", "Port Address"=w149) -> ("error out"=w143:errorcluster, "Response"=w140:string)  [unwired: 1 in, 3 out]
        n96 = call "Wait+.vi"("Error In"=w143, "milliseconds to wait"=u32 0) -> ("Error Out"=→"Error Out":errorcluster)  [unwired: 4 in, 1 out]
        n97 = Equal?(x=w140, y="103J012" ("Response")) -> (x = y?=w148:bool)
        n98 = Select(t="Connected" ("Response"), s=w148, f="Wrong Address" ("Response")) -> (s? t:f=→"Test Results":string)
        n99 = Not(x=w148) -> (.not. x?=w147:bool)
      }
      event "Run": Value Change {
        # "Move vi"
        n100 = event-data() -> ()  [unwired: 1 in, 6 out]
        n101 = property on="Parameter changed" class="Bool (strict)"("Val(Sgnl)"=TRUE ("Value (Signaling)")) -> ()  [unwired: 2 in, 2 out]
        n102 = local read "SPEED (rot/sec)\nincrement .0042"() -> (w168:dbl)
        n103 = In Range and Coerce(upper limit=0.42 ("x"), x=w168, lower limit=0.0042) -> (coerced(x)=w162:dbl)  [unwired: 1 out]
        n104 = Format Value(string ("")="VE", format string="%4.4", value (0)=w162) -> (output string=w158:string)
        n105 = local read "MODE:"() -> (w154:enum32{"ABSOLUTE", "INCREMENTAL"})
        n106 = Number To Boolean Array(number=w154) -> (Boolean array=w155:bool[])
        n107 = Index Array(array=w155) -> (element=w153:bool)  [unwired: 1 in]
        n108 = call "BLM Command.vi"("Motor Address"=w167, "Read Echo?"=FALSE, "Command"=w158, "Port Address"=w169) -> ("error out"=w166:errorcluster)  [unwired: 2 in, 4 out]
        n109 = call "BLM Move.vi"("Mode IS:"=w153, "Steps/rot"=w170, "error in (no error)"=w166, "Position / Distance"="New position", "Motor Address"=w167, "Port Address"=w169) -> ("error out"=w165:errorcluster)
        n110 = flat-sequence {
          tunnel: w165 -> [_]
          frame #0 {
            n111 = local write "Run"(FALSE ("Run")) -> ()
          }
        }
      }
    }
    n112 = Or(x=w25, y=FALSE) -> (x .or. y?=w26:bool)
  }
  n113 = property on="Test Connection" class="Bool"("Disabled"=w7) -> ()  [unwired: 2 in, 2 out]
  n114 = property on="Read Position" class="Bool"("Disabled"=w7) -> ()  [unwired: 2 in, 2 out]
  n115 = property on="Set Position" class="Bool"("Disabled"=w7) -> ()  [unwired: 2 in, 2 out]
  n116 = property on="SPEED (rot/sec)\nincrement .0042" class="DigNum (strict)"("Disabled"=w7) -> ()  [unwired: 2 in, 2 out]
  n117 = property on="New position" class="DigNum (strict)"("Disabled"=w7, "Value"=0.0 ("New position / \n distance (deg of BLM)"), "Caption.Text"=w14) -> ()  [unwired: 2 in, 2 out]
  n118 = Create User Event(user event datatype="") -> (user event=w3:refnum<user-event>)  [unwired: 1 in, 1 out]
  n119 = register-events(w3) -> (reference out=w5:refnum<event-registration>)  [unwired: 2 in, 1 out]
  n120 = call "stepper controller -- BLM.vi"("stepper driver action"=stepper_motor_action."init" ("stepper motor action")) -> ("stepper motor state OUT"=w1:T1)  [unwired: 8 in, 2 out]
  n121 = while {
    tunnel: w5 -> [w172]
    tunnel: w1 -> [_]
    stop <- _ stop-if-true
    n122 = event shown="[1] \"Run\": Value Change" {
      selector: w172 -> [_ _]
      dyn-events: _ -> [_ _]
      timeout: _ -> [_ _]
      event Timeout {
        n123 = event-data() -> ()  [unwired: 1 in, 3 out]
      }
      event "Run": Value Change {
        n124 = event-data() -> ()  [unwired: 1 in, 5 out]
        n125 = call "stepper controller -- BLM.vi"("stepper driver action"=stepper_motor_action."go" ("stepper motor action")) -> ()  [unwired: 8 in, 3 out]
      }
    }
  }
  n126 = while {
    tunnel: w1 -> [_]
    stop <- _ stop-if-true
    n127 = Wait Until Next ms Multiple(millisecond multiple=u32 100) -> ()  [unwired: 1 out]
    n128 = call "slider setter.vi"("slider setter action"=slider_setter_action."set current step") -> ()  [unwired: 10 in, 1 out]
  }
